vi "Пример графика интенсивности.vi"() -> ()   [LabVIEW 2017]
doc: "This VI is an exercise in the LabVIEW Basics I course.\n\nThis VI uses an intensity graph to plot an interference pattern, or a 2-D array of user-defined values. The intensity graph maps intensity values to colors. The intensity values are stored in a 2-D array. The row number of a value in the 2-D array corresponds to the location along the X-axis of the graph, and the column number corresponds to the location on the Y-axis."
panel:
  out "График интенсивности":dbl[][](graph)
  in  "График":bool
  in  "Данные пользователя":dbl[][](array[numeric])=[[10.0, 6.0, 7.0, 2.0], [3.0, 7.0, 4.0, 10.0], [1.0, 5.0, 10.0, 0.0], [7.0, 3.0, 1.0, 5.0]] format="%.2f"
  # "Данные пользователя"
  # "Интерференционная картина"
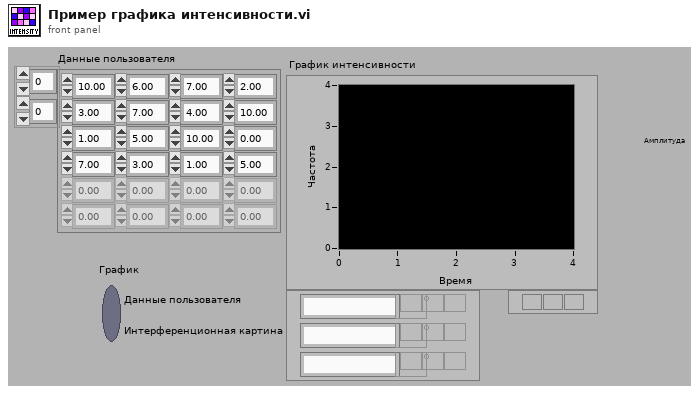
[diagram p1: front panel]
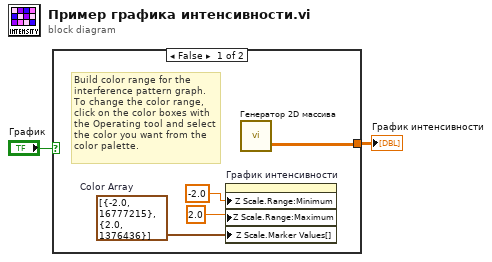
[diagram p0: block diagram]
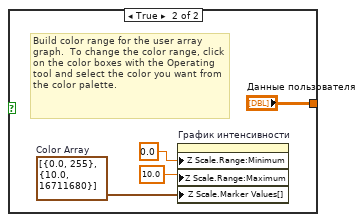
[diagram p2: hidden frame]
diagram:
  n1 = case shown="False" "График" {
    tunnel: [w5 "Данные пользователя"] -> w1
    frame False {
      w6 = cluster{dbl, u32}[] [{-2.0, 16777215}, {2.0, 1376436}]  # Color Array
      # "Build color range for the interference pattern graph.  To change the color range, click on the color boxes with the Operating tool and select the color you want from the color palette."
      n2 = property on="График интенсивности" class="IntGraph (strict)"("Z Scale.Range:Minimum"=-2.0, "Z Scale.Range:Maximum"=2.0, "Z Scale.Marker Values[]"=w6) -> ()  [unwired: 2 in, 2 out]
      n3 = call "Генератор 2D массива.vi"() -> ("data"=w5:dbl[][])  [unwired: 5 in, 1 out]
    }
    frame True {
      w7 = cluster{dbl, u32}[] [{0.0, 255}, {10.0, 16711680}]  # Color Array
      # "Build color range for the user array graph.  To change the color range, click on the color boxes with the Operating tool and select the color you want from the color palette."
      n4 = property on="График интенсивности" class="IntGraph (strict)"("Z Scale.Range:Minimum"=0.0, "Z Scale.Range:Maximum"=10.0, "Z Scale.Marker Values[]"=w7) -> ()  [unwired: 2 in, 2 out]
    }
  }
  "График интенсивности" <- w1
